vi "CLD 9 Step Sequencer Express Timer Front Panel.vi"() -> ()   [LabVIEW 2025]
doc: "CLD 9 Exercise"
panel:
  out "Current Step Time":dbl
  out "Elapsed Time (s)":string
  out "Step 3":bool
  out "Step 2":bool
  out "Step 1":bool
  out "Time Has Elapsed":bool
  in  "Auto Reset":bool=TRUE
  in  "Reset Button":bool
  in  "Stop VI":bool
  out "error out":errorcluster
  in  "error in (no error)":errorcluster
  in  "Time Target (s)":dbl
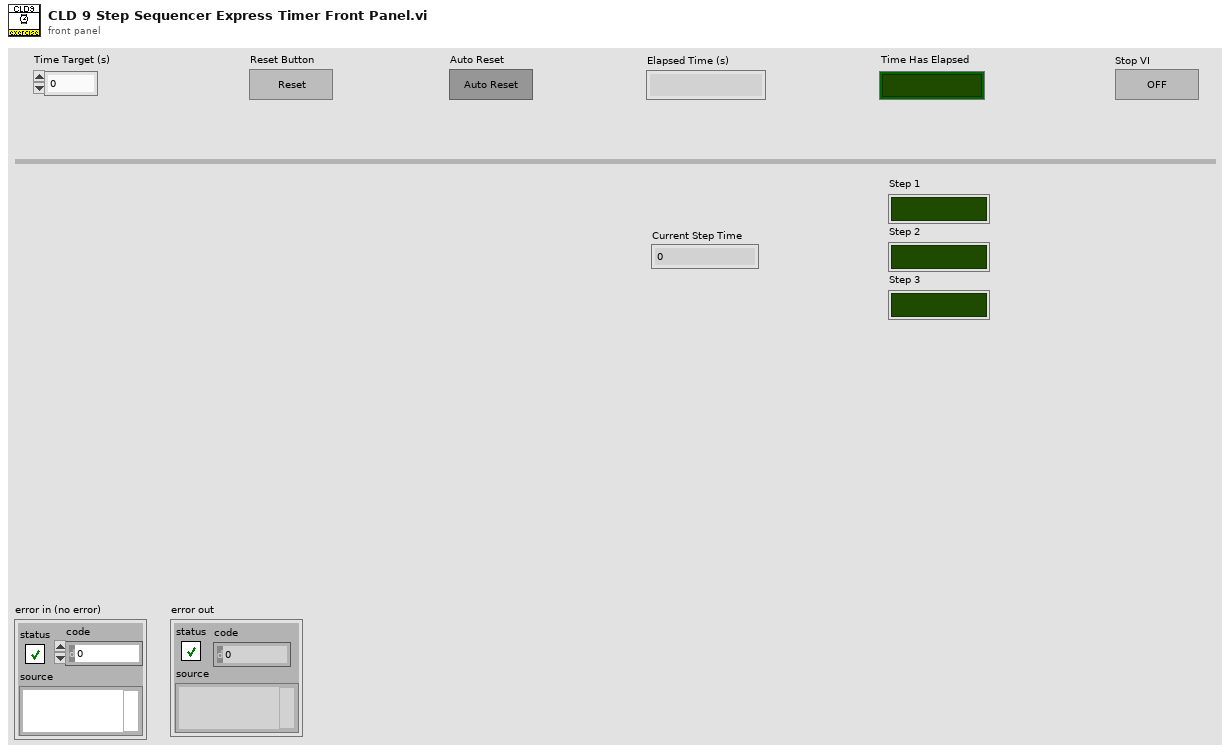
[diagram p1: front panel]
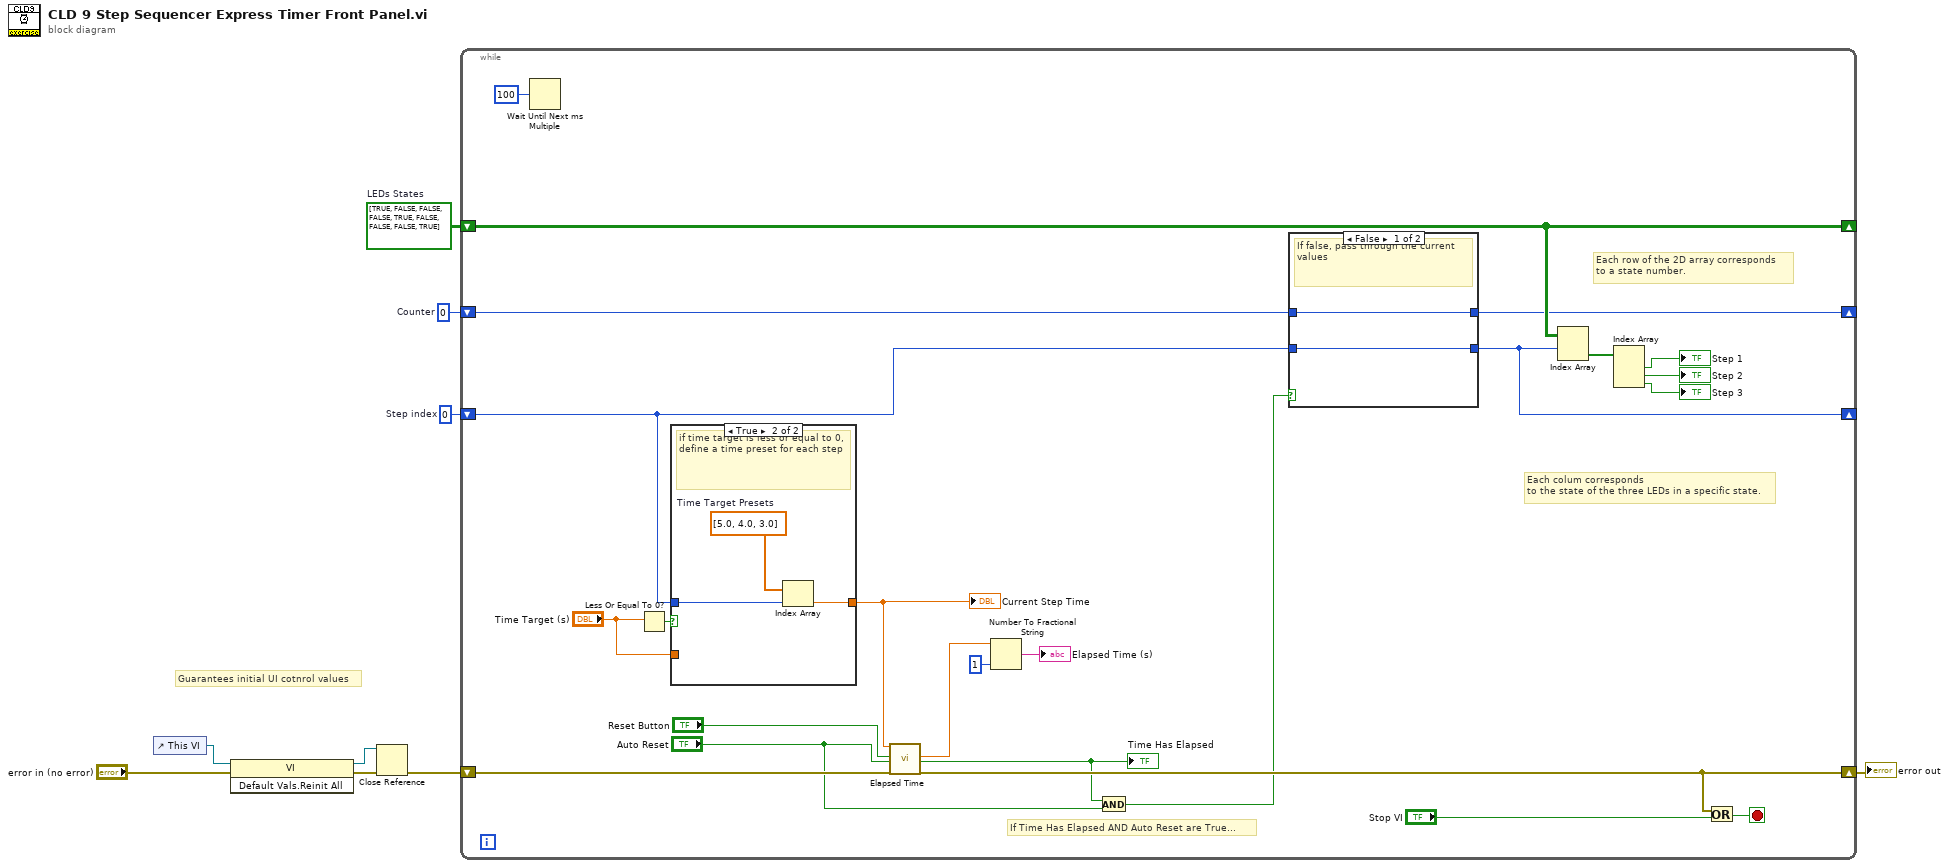
[diagram p0: block diagram]
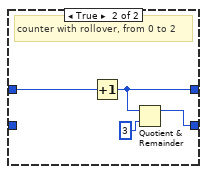
[diagram p3: hidden frame]
diagram:
  w5 = 0  # Step index
  w6 = 0  # Counter
  w7 = bool[][] [[TRUE, FALSE, FALSE], [FALSE, TRUE, FALSE], [FALSE, FALSE, TRUE]]  # LEDs States
  # "Guarantees initial UI cotnrol values"
  n1 = control-ref of="This VI"() -> (w3:refnum<vi>)
  n2 = invoke class="VI" method="Default Vals.Reinit All"(reference=w3, error in="error in (no error)") -> (reference out=w1:refnum<vi>, error out=w4:errorcluster)  [unwired: 1 in, 1 out]
  n3 = Close Reference(reference=w1, error in (no error)=w4) -> (error out=w2:errorcluster)
  n4 = while {
    shift-right: [w27] -> w8
    shift-left: w2 -> [w33]
    shift-right: [w25] -> _
    shift-left: w7 -> [w25]
    shift-right: [w23] -> _
    shift-left: w6 -> [w24]
    shift-right: [w15] -> _
    shift-left: w5 -> [w13]
    stop <- w28 stop-if-true
    # "Each row of the 2D array corresponds\nto a state number."
    # "Each colum corresponds\nto the state of the three LEDs in a specific state."
    # "If Time Has Elapsed AND Auto Reset are True..."
    n5 = Wait Until Next ms Multiple(millisecond multiple=u32 100) -> ()  [unwired: 1 out]
    n6 = Less Or Equal To 0?(x="Time Target (s)") -> (x <= 0?=w14:bool)
    n7 = case shown="True" w14 {
      tunnel: w13 -> [_ w36]
      tunnel: [w34 w35] -> w12
      tunnel: "Time Target (s)" -> [w34 _]
      frame False {
      }
      frame True {
        w37 = dbl[] [5.0, 4.0, 3.0]  # Time Target Presets
        # "if time target is less or equal to 0, define a time preset for each step"
        n8 = Index Array(array=w37, index=w36) -> (element=w35:dbl)
      }
    }
    "Current Step Time" <- w12
    n9 = call "Elapsed Time"("Time Target (s)"=w12, "Reset"="Reset Button", "Auto Reset"="Auto Reset", "error in (no error)"=w33) -> ("Elapsed Time (s)"=w31:dbl, "Time has Elapsed"=w18:bool, "error out"=w27:errorcluster)  [unwired: 8 in, 5 out]
    "Time Has Elapsed" <- w18
    n10 = Number To Fractional String(number=w31, precision (6)=i16 1) -> (F-format string=→"Elapsed Time (s)":string)  [unwired: 2 in]
    n11 = And(x=w18, y="Auto Reset") -> (x .and. y?=w17:bool)
    n12 = case shown="False" w17 {
      tunnel: [w38 w42] -> w15
      tunnel: w24 -> [w39 w41]
      tunnel: [w39 w40] -> w23
      tunnel: w13 -> [w38 _]
      frame False {
        # "If false, pass through the current values"
      }
      frame True {
        # "counter with rollover, from 0 to 2"
        n13 = Increment(x=w41) -> (x+1=w40:i32)
        n14 = Quotient & Remainder(x=w40, y=3) -> (x-y*floor(x/y)=w42:i32)  [unwired: 1 out]
      }
    }
    n15 = Index Array(array=w25, index (row)=w15) -> (element=w22:bool[])  [unwired: 1 in]
    n16 = Index Array(array=w22) -> (element #1=→"Step 1":bool, element #2=→"Step 2":bool, element #3=→"Step 3":bool)  [unwired: 3 in]
    n17 = Or(x=w27, y="Stop VI") -> (x .or. y?=w28:bool)
  }
  "error out" <- w8
